vi "Hardware Device Get Info.vi"(8 "error in":errorcluster, 11 "NI Digital Input in":refnum<class "NI Digital Input.lvclass">) -> (0 "error out":errorcluster, 3 "NI Digital Input out":refnum<class "NI Digital Input.lvclass">)   [LabVIEW 2023, in "HardwareAbstractionLayer_LVOOP.lvlib" / "NI Digital Input.lvclass"]
doc: "This VI is AI Physical Channel Read"
uses:
  NI Digital Input.lvclass
  NI Digital Input.lvclass/NI Digital Input.ctl
  <resource>/objmgr/daqmx.rc
  Teststand/Teststand.lvclass
panel:
  out "DI.Lines":tag[](array[tag])
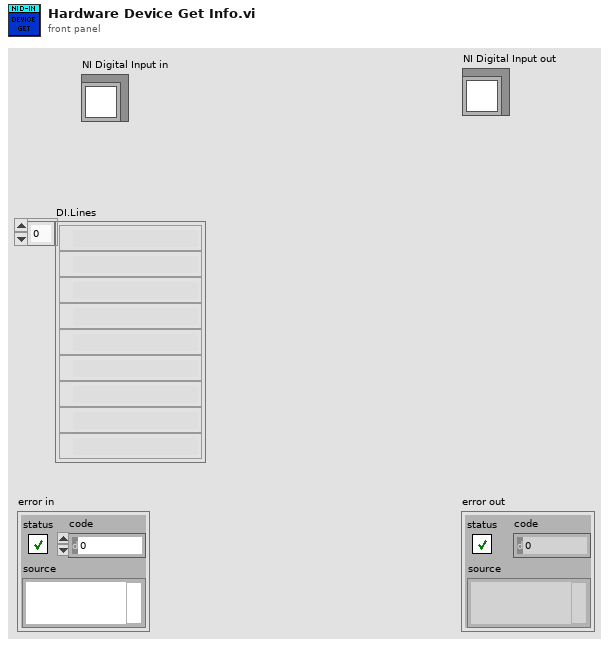
[diagram p1: front panel]
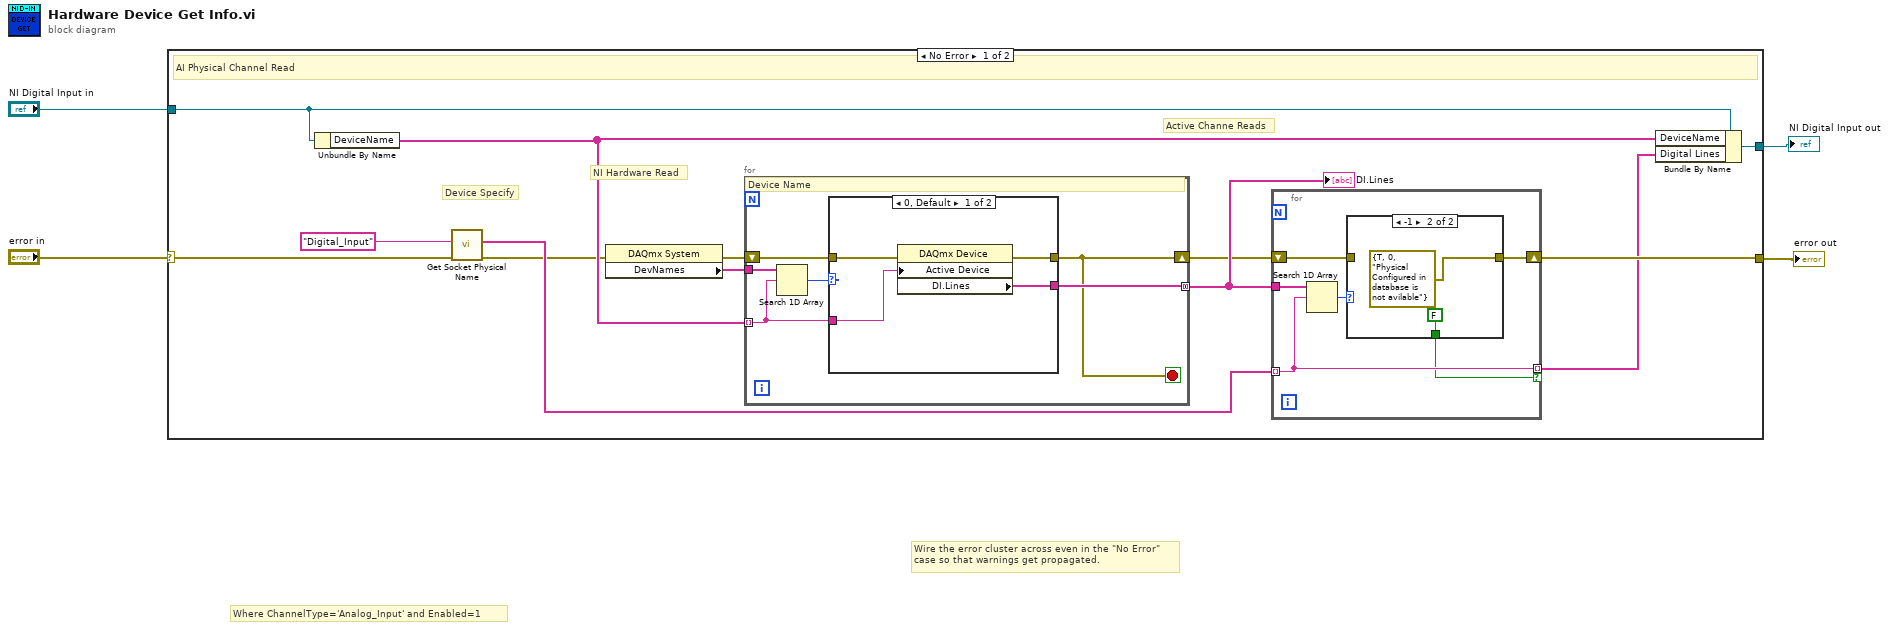
[diagram p0: block diagram]
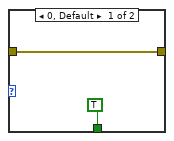
[diagram p2: hidden frame]
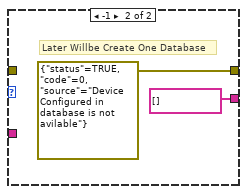
[diagram p3: hidden frame]
diagram:
  # "Where ChannelType='Analog_Input' and Enabled=1"
  # "Wire the error cluster across even in the \"No Error\"\ncase so that warnings get propagated."
  n1 = case shown="No Error" "error in" {
    selector: "error in" -> [w6 w41]
    tunnel: [w10 w41] -> w3
    tunnel: [w17 w40] -> w1
    tunnel: "NI Digital Input in" -> [w16 w40]
    frame No Error {
      # "Active Channe Reads"
      # "Device Specify"
      # "NI Hardware Read"
      # "AI Physical Channel Read"
      n2 = Unbundle By Name(w16) -> ("DeviceName"=w15:tag[])
      n3 = call "Get Socket Physical Name.vi"("error In"=w6, "ChannelType"="Digital_Input") -> ("error out"=w7:errorcluster, "Physical Channel"=w8:tag[])  [unwired: 7 in, 1 out]
      n4 = property class="DAQmx System"(error in=w7) -> (error out=w13:errorcluster, "DevNames"=w14:tag[])  [unwired: 1 in, 1 out]
      n5 = for {
        tunnel: w15 -> [w30] mode=indexing
        tunnel: w14 -> [w31]
        tunnel: [w29] -> w12 mode=concatenating
        shift-right: [w28] -> w11
        shift-left: w13 -> [w32]
        stop <- w28 stop-if-true
        # "Device Name"
        n6 = Search 1D Array(1D array=w31, element=w30) -> (index of element=w33:i32)  [unwired: 1 in]
        n7 = case shown="0, Default" w33 {
          tunnel: w32 -> [w35 _]
          tunnel: [w34 errorcluster {"status"=TRUE, "code"=0, "source"="Device  Configured in database is not avilable"} ("error out")] -> w28
          tunnel: w30 -> [w37 _]
          tunnel: [w36 tag[] [] ("AI.PhysicalChans")] -> w29
          frame 0, Default {
            n8 = property class="DAQmx Device"(error in=w35, "Active Device"=w37) -> (error out=w34:errorcluster, "DI.Lines"=w36:tag[])  [unwired: 1 in, 1 out]
          }
          frame -1 {
            # "Later Willbe Create One Database"
          }
        }
      }
      "DI.Lines" <- w12
      n9 = for {
        tunnel: w12 -> [w23]
        tunnel: w8 -> [w19] mode=indexing
        shift-right: [w20] -> w10
        shift-left: w11 -> [w21]
        tunnel: [w19] -> w9 mode=indexing if=w18
        n10 = Search 1D Array(1D array=w23, element=w19) -> (index of element=w22:i32)  [unwired: 1 in]
        n11 = case shown="-1" w22 {
          tunnel: w21 -> [w25 _]
          tunnel: [w25 errorcluster {"status"=TRUE, "code"=0, "source"="Physical Configured in database is not avilable"} ("error out")] -> w20
          tunnel: [TRUE FALSE] -> w18
          frame 0, Default {
          }
          frame -1 {
          }
        }
      }
      n12 = Bundle By Name(cluster=w16, "DeviceName"=w15, "Digital Lines"=w9) -> (w17:refnum<class "NI Digital Input.lvclass">)
    }
    frame Error {
    }
  }
  "error out" <- w3
  "NI Digital Input out" <- w1
